vi "LB_FocusIndexArray_Tests.vi"(11 "error in":errorcluster) -> (15 "error out":errorcluster)   [LabVIEW 2016, in "DronaTest.lvlib"]
uses:
  DronaTest.lvlib
  APIs/Stimulus/ControlValue/SetValueAuto.vi
  APIs/Stimulus/ControlValue/Controls/Listbox/SetValueByArrayIndex.vi
  APIs/Assert/AssertControlValue/Controls/Listbox/AssertValueByArrayIndex.vi
  <vilib>/addons/_JKI Toolkits/Caraya/classes/Assert/Assert Error.vi
  <vilib>/addons/_JKI Toolkits/Caraya/classes/Assert/Assert Equal Value_Variant.vi
  <vilib>/addons/_JKI Toolkits/Caraya/classes/Test/Test.lvclass
  Drona.lvlib
  <vilib>/SLL Toolkit/SLL Debug/SLL Debug.lvlib
  APIs/Stimulus/ControlValue/ControlValue.lvlib
  <vilib>/addons/_JKI Toolkits/Caraya/classes/Assert/Assert.lvclass
  APIs/Stimulus/ControlValue/Controls/Listbox/StimulusListbox.lvlib
  APIs/Assert/AssertControlValue/Controls/Listbox/AssertListbox.lvlib
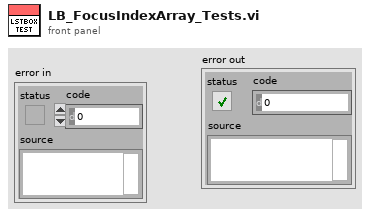
[diagram p1: front panel]
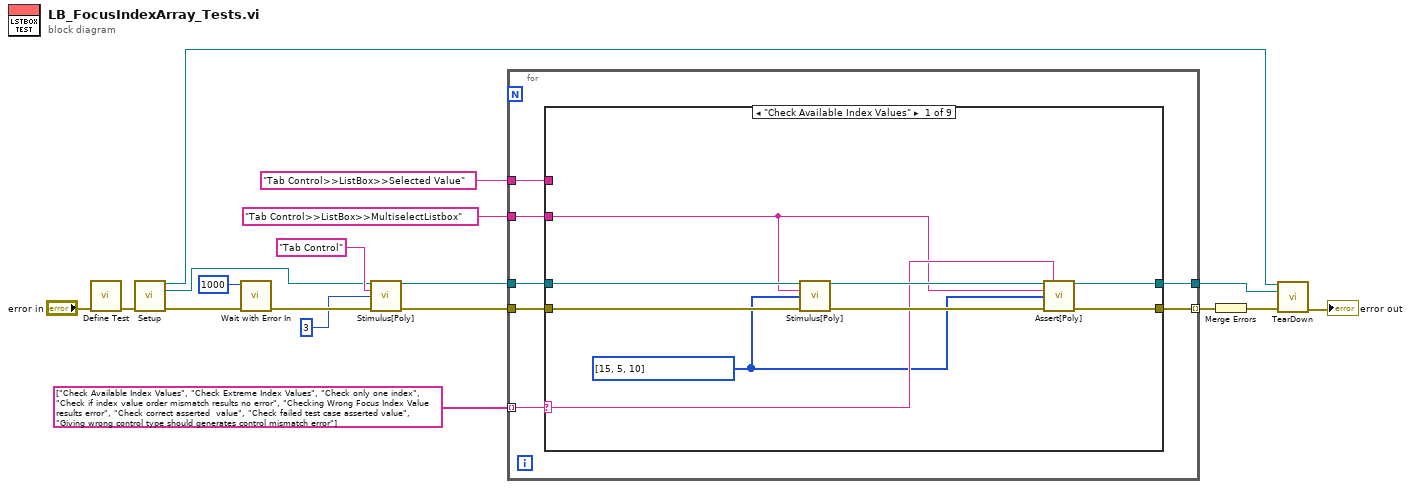
[diagram p0: block diagram]
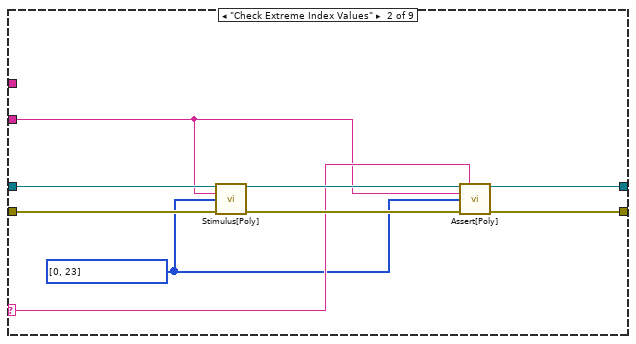
[diagram p2: hidden frame]
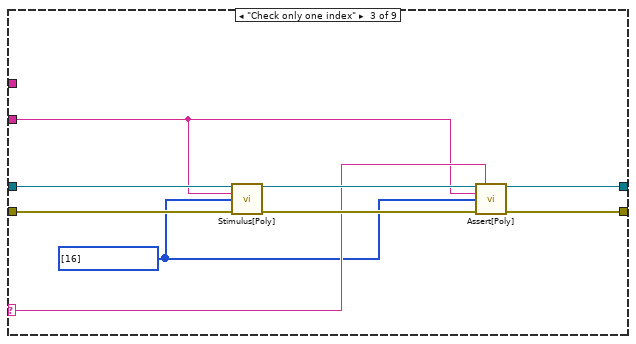
[diagram p3: hidden frame]
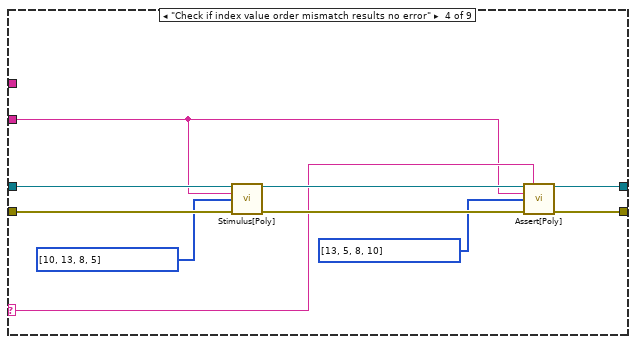
[diagram p4: hidden frame]
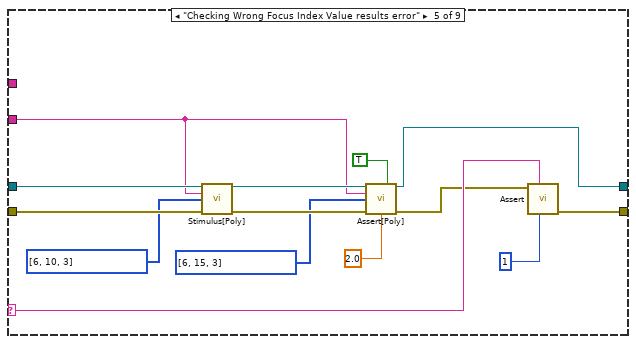
[diagram p5: hidden frame]
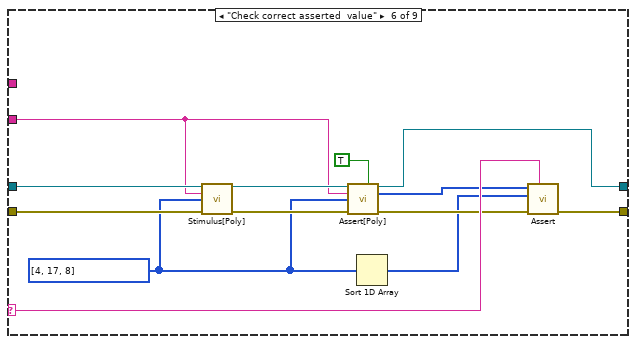
[diagram p6: hidden frame]
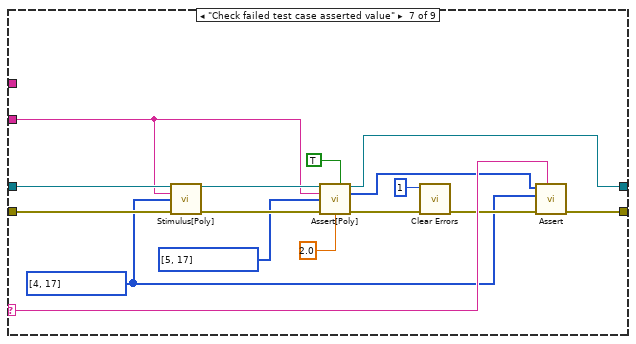
[diagram p7: hidden frame]
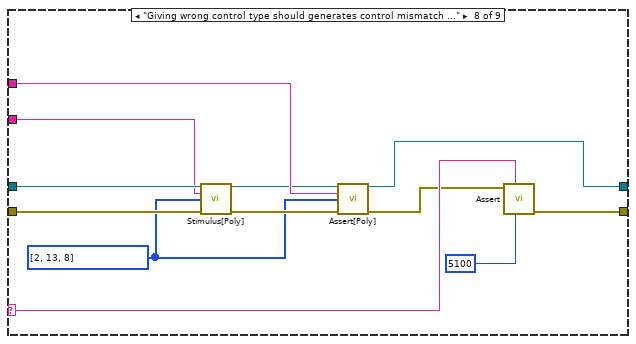
[diagram p8: hidden frame]
diagram:
  n1 = call <vilib>:"Define Test.vi"("error in (no error)"="error in") -> ("error out"=w7:errorcluster)  [unwired: 10 in]
  n2 = call "Setup.vi"("error in (no error)"=w7) -> ("Application Ref"=w3:refnum<vi>, "VI out"=w5:refnum<vi>, "error out"=w6:errorcluster)  [unwired: 12 in]
  n3 = call <vilib>:"Wait with Error In.vi"("error in (no error)"=w6, "milliseconds to wait"=u32 1000) -> ("error out"=w16:errorcluster)  [unwired: 9 in]
  n4 = call-poly "Stimulus[Poly].vi"("VI Reference In"=w5, "Control Path"="Tab Control", "Value (Signaling)"=3, "error in"=w16) -> ("VI Reference Out"=w12:refnum<vi>, "error out"=w15:errorcluster)  [unwired: 10 in]
  n5 = for {
    tunnel: w12 -> [w24]
    tunnel: "Tab Control>>ListBox>>MultiselectListbox" ("Control Path") -> [w23]
    tunnel: "Tab Control>>ListBox>>Selected Value" ("Control Path") -> [w22]
    tunnel: string[] ["Check Available Index Values", "Check Extreme Index Values", "Check only one index", "Check if index value order mismatch results no error", "Checking Wrong Focus Index Value results error", "Check correct asserted  value", "Check failed test case asserted value", "Giving wrong control type should generates control mismatch error"] -> [w20] mode=indexing
    tunnel: [w19] -> w2
    tunnel: w15 -> [w25]
    tunnel: [w21] -> w8 mode=indexing
    n6 = case shown="\"Check Available Index Values\"" w20 {
      selector: w20 -> [w28 w37 w46 w56 w75 w88 w104 w116 _]
      tunnel: w25 -> [w34 w43 w52 w62 w73 w87 w103 w111 w119]
      tunnel: w24 -> [w33 w42 w51 w61 w72 w86 w102 w109 w118]
      tunnel: w23 -> [w27 w36 w45 w55 w69 w83 w99 w107 _]
      tunnel: w22 -> [_ _ _ _ _ _ _ w113 _]
      tunnel: [w30 w39 w48 w58 w76 w89 w105 w117 w119] -> w21
      tunnel: [w29 w38 w47 w57 w68 w82 w98 w112 w118] -> w19
      frame "Check Available Index Values" {
        w26 = i32[] [15, 5, 10] ("Index Array")
        n7 = call-poly "Stimulus[Poly].vi"("VI Reference In"=w33, "Control Path"=w27, "Index Array"=w26, "Error In"=w34) -> ("VI Reference Out"=w31:refnum<vi>, "Error Out"=w32:errorcluster)  [unwired: 10 in]
        n8 = call-poly "Assert[Poly].vi"("VI Reference In"=w31, "Test Label"=w28, "Control Path"=w27, "Focus Item Index"=w26, "Error In"=w32) -> ("VI Reference Out"=w29:refnum<vi>, "Error Out"=w30:errorcluster)  [unwired: 8 in, 1 out]
      }
      frame "Check Extreme Index Values" {
        w35 = i32[] [0, 23] ("Index Array")
        n9 = call-poly "Stimulus[Poly].vi"("VI Reference In"=w42, "Control Path"=w36, "Index Array"=w35, "Error In"=w43) -> ("VI Reference Out"=w40:refnum<vi>, "Error Out"=w41:errorcluster)  [unwired: 10 in]
        n10 = call-poly "Assert[Poly].vi"("VI Reference In"=w40, "Test Label"=w37, "Control Path"=w36, "Focus Item Index"=w35, "Error In"=w41) -> ("VI Reference Out"=w38:refnum<vi>, "Error Out"=w39:errorcluster)  [unwired: 8 in, 1 out]
      }
      frame "Check only one index" {
        w44 = i32[] [16] ("Index Array")
        n11 = call-poly "Stimulus[Poly].vi"("VI Reference In"=w51, "Control Path"=w45, "Index Array"=w44, "Error In"=w52) -> ("VI Reference Out"=w49:refnum<vi>, "Error Out"=w50:errorcluster)  [unwired: 10 in]
        n12 = call-poly "Assert[Poly].vi"("VI Reference In"=w49, "Test Label"=w46, "Control Path"=w45, "Focus Item Index"=w44, "Error In"=w50) -> ("VI Reference Out"=w47:refnum<vi>, "Error Out"=w48:errorcluster)  [unwired: 8 in, 1 out]
      }
      frame "Check if index value order mismatch results no error" {
        n13 = call-poly "Stimulus[Poly].vi"("VI Reference In"=w61, "Control Path"=w55, "Index Array"=i32[] [10, 13, 8, 5], "Error In"=w62) -> ("VI Reference Out"=w59:refnum<vi>, "Error Out"=w60:errorcluster)  [unwired: 10 in]
        n14 = call-poly "Assert[Poly].vi"("VI Reference In"=w59, "Test Label"=w56, "Control Path"=w55, "Focus Item Index"=i32[] [13, 5, 8, 10] ("Index Array"), "Error In"=w60) -> ("VI Reference Out"=w57:refnum<vi>, "Error Out"=w58:errorcluster)  [unwired: 8 in, 1 out]
      }
      frame "Checking Wrong Focus Index Value results error" {
        n15 = call-poly "Stimulus[Poly].vi"("VI Reference In"=w72, "Control Path"=w69, "Index Array"=i32[] [6, 10, 3], "Error In"=w73) -> ("VI Reference Out"=w70:refnum<vi>, "Error Out"=w71:errorcluster)  [unwired: 10 in]
        n16 = call-poly "Assert[Poly].vi"("VI Reference In"=w70, "Assert Only? (F)"=TRUE, "Control Path"=w69, "Focus Item Index"=i32[] [6, 15, 3] ("Index Array"), "Error In"=w71, "Timeout(5 sec)"=2.0) -> ("VI Reference Out"=w68:refnum<vi>, "Error Out"=w67:errorcluster)  [unwired: 7 in, 1 out]
        n17 = call-poly <vilib>:"Assert.vi"("error code (1)"=1, "Label"=w75, "Error?"=w67) -> ("error out"=w76:errorcluster)  [unwired: 8 in]
      }
      frame "Check correct asserted  value" {
        w78 = i32[] [4, 17, 8] ("Index Array")
        n18 = call-poly "Stimulus[Poly].vi"("VI Reference In"=w86, "Control Path"=w83, "Index Array"=w78, "Error In"=w87) -> ("VI Reference Out"=w84:refnum<vi>, "Error Out"=w85:errorcluster)  [unwired: 10 in]
        n19 = call-poly "Assert[Poly].vi"("VI Reference In"=w84, "Assert Only? (F)"=TRUE, "Control Path"=w83, "Focus Item Index"=w78, "Error In"=w85) -> ("VI Reference Out"=w82:refnum<vi>, "Asserted Value"=w80:i32[], "Error Out"=w81:errorcluster)  [unwired: 8 in]
        n20 = Sort 1D Array(array=w78) -> (sorted array=w77:i32[])
        n21 = call-poly <vilib>:"Assert.vi"("Label"=w88, "error in (no error)"=w81, "Y"=w77, "X"=w80) -> ("error out"=w89:errorcluster)  [unwired: 7 in]
      }
      frame "Check failed test case asserted value" {
        w91 = i32[] [4, 17] ("Index Array")
        n22 = call-poly "Stimulus[Poly].vi"("VI Reference In"=w102, "Control Path"=w99, "Index Array"=w91, "Error In"=w103) -> ("VI Reference Out"=w100:refnum<vi>, "Error Out"=w101:errorcluster)  [unwired: 10 in]
        n23 = call-poly "Assert[Poly].vi"("VI Reference In"=w100, "Assert Only? (F)"=TRUE, "Control Path"=w99, "Focus Item Index"=i32[] [5, 17] ("Index Array"), "Error In"=w101, "Timeout(5 sec)"=2.0) -> ("VI Reference Out"=w98:refnum<vi>, "Asserted Value"=w92:i32[], "Error Out"=w97:errorcluster)  [unwired: 7 in]
        n24 = call <vilib>:"Clear Errors.vi"("error in (no error)"=w97, "specific error code to clear (0: all)"=1) -> ("error out"=w94:errorcluster)  [unwired: 4 in, 1 out]
        n25 = call-poly <vilib>:"Assert.vi"("Label"=w104, "error in (no error)"=w94, "Y"=w91, "X"=w92) -> ("error out"=w105:errorcluster)  [unwired: 7 in]
      }
      frame "Giving wrong control type should generates control mismatch error" {
        w106 = i32[] [2, 13, 8] ("Index Array")
        n26 = call-poly "Stimulus[Poly].vi"("VI Reference In"=w109, "Control Path"=w107, "Index Array"=w106, "Error In"=w111) -> ("VI Reference Out"=w108:refnum<vi>, "Error Out"=w110:errorcluster)  [unwired: 10 in]
        n27 = call-poly "Assert[Poly].vi"("VI Reference In"=w108, "Control Path"=w113, "Focus Item Index"=w106, "Error In"=w110) -> ("VI Reference Out"=w112:refnum<vi>, "Error Out"=w114:errorcluster)  [unwired: 9 in, 1 out]
        n28 = call-poly <vilib>:"Assert.vi"("error code (1)"=5100, "Label"=w116, "Error?"=w114) -> ("error out"=w117:errorcluster)  [unwired: 8 in]
      }
      frame Default {
      }
    }
  }
  n29 = Merge Errors(w8) -> (w4:errorcluster)
  n30 = call "TearDown.vi"("Application Ref"=w3, "VI in"=w2, "error in (no error)"=w4) -> ("error out"=→"error out":errorcluster)  [unwired: 12 in]
